vi "MakeThetaLabels.vi"(1 "ticsAndGrids":T1={"tics"={"ticMin"=0.0, "ticStep"=0.0, "ticMax"=0.0, "minorDivsPerMajor"=2, "ticSpacing"=enum."Auto Tics", "ticPosition"=enum."Inside, no mirror"}, "Grids"={"Gridlines"=enum."Major grid", "Zeroaxis"=enum."No zero axis"}, "Mapping"=enum."Lin"}) -> (0 "Theta Label Command String":string[](array[string]))   [LabVIEW 2015]
uses:
  ticsAndGrids.ctl
  tics.ctl
  grids.ctl
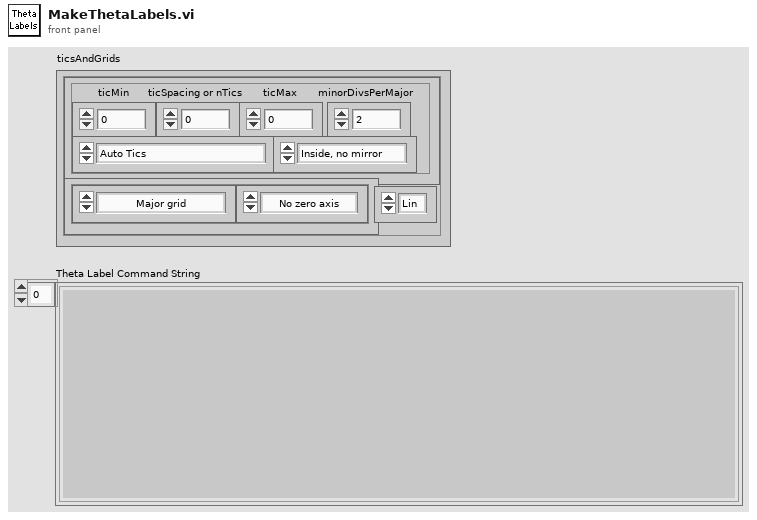
[diagram p1: front panel]
types:
  T1 = typedef "ticsAndGrids.ctl" = cluster{"tics":T2, "Grids":T3, "Mapping":enum8{"Lin", "Log"}}
  T2 = typedef "tics.ctl" = cluster{"ticMin":dbl, "ticStep":dbl, "ticMax":dbl, "minorDivsPerMajor":i32, "ticSpacing":enum16{"Auto Tics", "Fixed spacing", "Fixed Minimum and Spacing", "Start, Spacing and Maximum", "Approx n Tics (rounded)"}, "ticPosition":enum16{"Inside, no mirror", "Inside, mirrored", "Outside, no mirror", "Outside, mirrored", "Invisible"}}
  T3 = typedef "grids.ctl" = cluster{"Gridlines":enum16{"No grids", "Major grid", "Minor grid", "Major and Minor"}, "Zeroaxis":enum16{"No zero axis", "Show zero axis"}}
  T4 = enum16{"Auto Tics", "Fixed spacing", "Fixed Minimum and Spacing", "Start, Spacing and Maximum", "Approx n Tics (rounded)"}
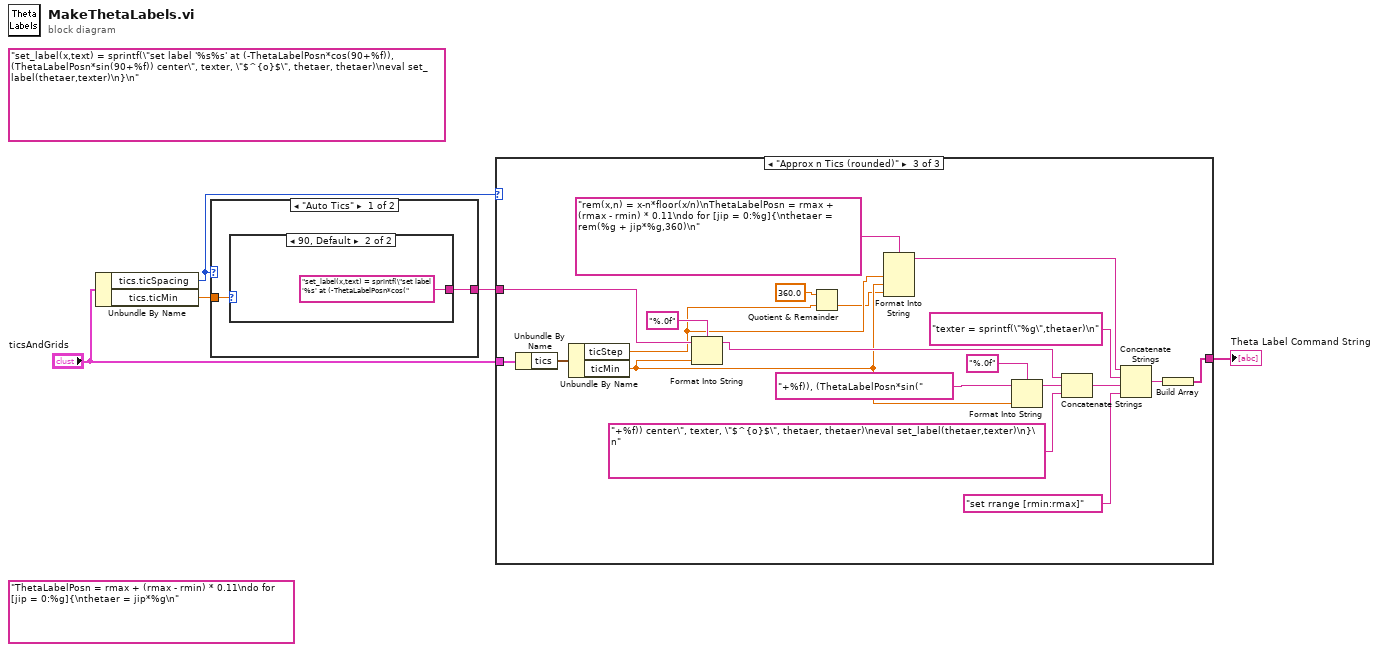
[diagram p0: block diagram]
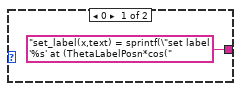
[diagram p2: hidden frame]
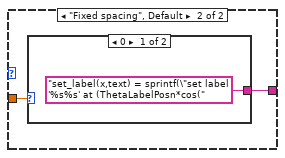
[diagram p3: hidden frame]
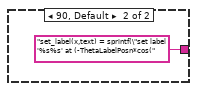
[diagram p4: hidden frame]
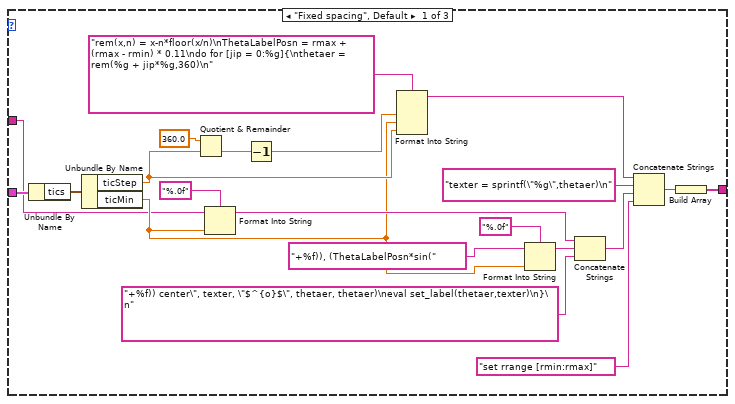
[diagram p5: hidden frame]
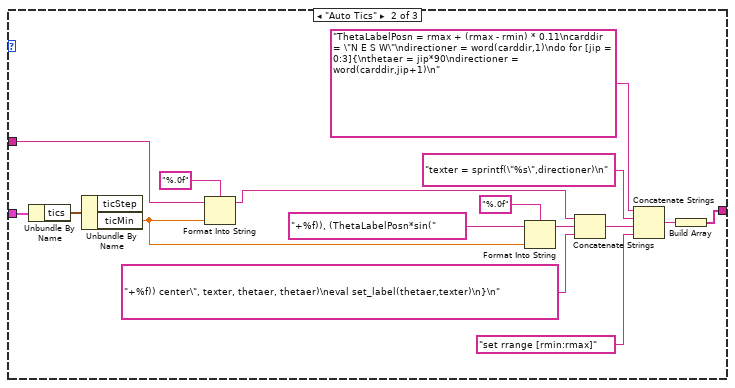
[diagram p6: hidden frame]
diagram:
  (unwired) "ThetaLabelPosn = rmax + (rmax - rmin) * 0.11\ndo for [jip = 0:%g]{\nthetaer = jip*%g\n"
  (unwired) "set_label(x,text) = sprintf(\"set label '%s%s' at (-ThetaLabelPosn*cos(90+%f)), (ThetaLabelPosn*sin(90+%f)) center\", texter, \"$^{o}$\", thetaer, thetaer)\neval set_label(thetaer,texter)\n}\n"
  n1 = Unbundle By Name("ticsAndGrids") -> ("tics.ticSpacing"=w1:T4, "tics.ticMin"=w3:dbl)
  n2 = case shown="\"Auto Tics\"" w1 {
    tunnel: w3 -> [w7 w11]
    tunnel: [w6 w10] -> w2
    frame "Auto Tics" {
      n3 = case shown="90, Default" w7 {
        tunnel: ["set_label(x,text) = sprintf(\"set label '%s' at (ThetaLabelPosn*cos(" "set_label(x,text) = sprintf(\"set label '%s' at (-ThetaLabelPosn*cos("] -> w6
        frame 0 {
        }
        frame 90, Default {
        }
      }
    }
    frame "Fixed spacing", Default {
      n4 = case shown="0" w11 {
        tunnel: ["set_label(x,text) = sprintf(\"set label '%s%s' at (ThetaLabelPosn*cos(" "set_label(x,text) = sprintf(\"set label '%s%s' at (-ThetaLabelPosn*cos("] -> w10
        frame 0 {
        }
        frame 90, Default {
        }
      }
    }
  }
  n5 = case shown="\"Approx n Tics (rounded)\"" w1 {
    tunnel: "ticsAndGrids" -> [w17 w38 w57]
    tunnel: [w16 w37 w56] -> w4
    tunnel: w2 -> [w14 w35 w54]
    frame "Fixed spacing", Default {
      n6 = Unbundle By Name(w17) -> ("tics"=w27:T2)
      n7 = Unbundle By Name(w27) -> ("ticStep"=w32:dbl, "ticMin"=w15:dbl)
      n8 = Quotient & Remainder(x=360.0, y=w32) -> (floor(x/y)=w29:dbl)  [unwired: 1 out]
      n9 = Format Into String(format string="%.0f", initial string=w14, w15) -> (resulting string=w21:string)  [unwired: 1 in, 1 out]
      n10 = Decrement(x=w29) -> (x-1=w31:dbl)
      n11 = Format Into String(format string="rem(x,n) = x-n*floor(x/n)\nThetaLabelPosn = rmax + (rmax - rmin) * 0.11\ndo for [jip = 0:%g]{\nthetaer = rem(%g + jip*%g,360)\n", w31, w15, w32) -> (resulting string=w33:string)  [unwired: 2 in, 1 out]
      n12 = Format Into String(format string="%.0f", initial string="+%f)), (ThetaLabelPosn*sin(", w15) -> (resulting string=w20:string)  [unwired: 1 in, 1 out]
      n13 = Concatenate Strings(w21, w20, "+%f)) center\", texter, \"$^{o}$\", thetaer, thetaer)\neval set_label(thetaer,texter)\n}\n") -> (w18:string)
      n14 = Concatenate Strings(w33, "texter = sprintf(\"%g\",thetaer)\n" ("string"), w18, "set rrange [rmin:rmax]" ("string")) -> (w26:string)
      n15 = Build Array(w26) -> (w16:string[])
    }
    frame "Auto Tics" {
      n16 = Unbundle By Name(w38) -> ("tics"=w49:T2)
      n17 = Unbundle By Name(w49) -> ("ticMin"=w39:dbl)  [unwired: 1 out]
      n18 = Format Into String(format string="%.0f", initial string=w35, w39) -> (resulting string=w43:string)  [unwired: 1 in, 1 out]
      n19 = Format Into String(format string="%.0f", initial string="+%f)), (ThetaLabelPosn*sin(", w39) -> (resulting string=w42:string)  [unwired: 1 in, 1 out]
      n20 = Concatenate Strings(w43, w42, "+%f)) center\", texter, thetaer, thetaer)\neval set_label(thetaer,texter)\n}\n") -> (w40:string)
      n21 = Concatenate Strings("ThetaLabelPosn = rmax + (rmax - rmin) * 0.11\ncarddir = \"N E S W\"\ndirectioner = word(carddir,1)\ndo for [jip = 0:3]{\nthetaer = jip*90\ndirectioner = word(carddir,jip+1)\n", "texter = sprintf(\"%s\",directioner)\n" ("string"), w40, "set rrange [rmin:rmax]" ("string")) -> (w48:string)
      n22 = Build Array(w48) -> (w37:string[])
    }
    frame "Approx n Tics (rounded)" {
      n23 = Unbundle By Name(w57) -> ("tics"=w67:T2)
      n24 = Unbundle By Name(w67) -> ("ticStep"=w53:dbl, "ticMin"=w55:dbl)
      n25 = Format Into String(format string="%.0f", initial string=w54, w55) -> (resulting string=w61:string)  [unwired: 1 in, 1 out]
      n26 = Quotient & Remainder(x=360.0, y=w53) -> (floor(x/y)=w51:dbl)  [unwired: 1 out]
      n27 = Format Into String(format string="rem(x,n) = x-n*floor(x/n)\nThetaLabelPosn = rmax + (rmax - rmin) * 0.11\ndo for [jip = 0:%g]{\nthetaer = rem(%g + jip*%g,360)\n", w53, w55, w51) -> (resulting string=w69:string)  [unwired: 2 in, 1 out]
      n28 = Format Into String(format string="%.0f", initial string="+%f)), (ThetaLabelPosn*sin(", w55) -> (resulting string=w60:string)  [unwired: 1 in, 1 out]
      n29 = Concatenate Strings(w61, w60, "+%f)) center\", texter, \"$^{o}$\", thetaer, thetaer)\neval set_label(thetaer,texter)\n}\n") -> (w58:string)
      n30 = Concatenate Strings(w69, "texter = sprintf(\"%g\",thetaer)\n" ("string"), w58, "set rrange [rmin:rmax]" ("string")) -> (w66:string)
      n31 = Build Array(w66) -> (w56:string[])
    }
  }
  "Theta Label Command String" <- w4
